vi "TypedescToEnum.vi"(1 "type desc":i16[](array[numeric])) -> (0 "DataType":u16)   [LabVIEW 2010]
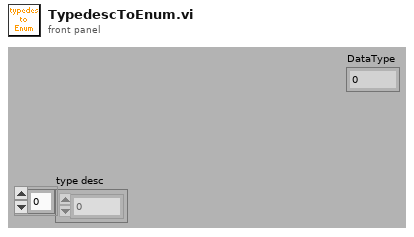
[diagram p1: front panel]
types:
  T1 = enum16{"I8", "I16", "I32", "U8", "U16", "U32", "SGL", "DBL", "Boolean", "String", "Array1D(I8)", "Array1D(I16)", "Array1D(I32)", "Array1D(U8)", "Array1D(U16)", "Array1D(U32)", "Array1D(SGL)", "Array1D(DBL)", "Array1D(Boolean)", "Array1D(String)", "Array2D(I8)", "Array2D(I16)", "Array2D(I32)", "Array2D(U8)", "Array2D(U16)", "Array2D(U32)", "Array2D(SGL)", "Array2D(DBL)", "Array2D(Boolean)", "Array2D(String)"}
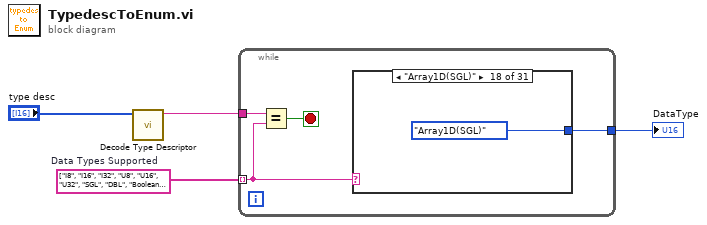
[diagram p0: block diagram]
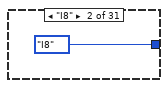
[diagram p3: hidden frame]
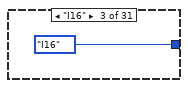
[diagram p4: hidden frame]
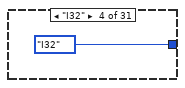
[diagram p5: hidden frame]
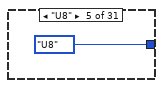
[diagram p6: hidden frame]
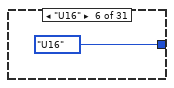
[diagram p7: hidden frame]
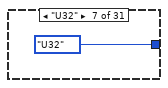
[diagram p8: hidden frame]
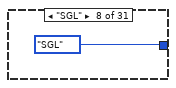
[diagram p9: hidden frame]
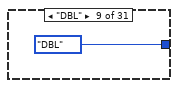
[diagram p10: hidden frame]
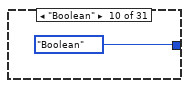
[diagram p11: hidden frame]
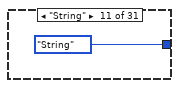
[diagram p12: hidden frame]
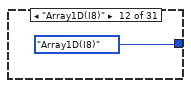
[diagram p13: hidden frame]
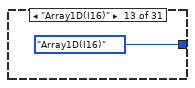
[diagram p14: hidden frame]
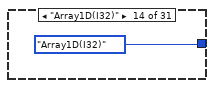
[diagram p15: hidden frame]
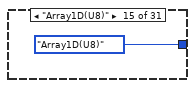
[diagram p16: hidden frame]
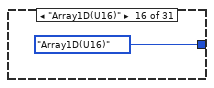
[diagram p17: hidden frame]
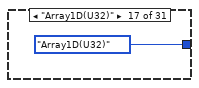
[diagram p18: hidden frame]
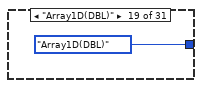
[diagram p19: hidden frame]
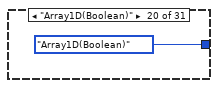
[diagram p20: hidden frame]
diagram:
  w3 = string[] ["I8", "I16", "I32", "U8", "U16", "U32", "SGL", "DBL", "Boolean", "String", "Array1D(I8)", "Array1D(I16)", "Array1D(I32)", "Array1D(U8)", "Array1D(U16)", "Array1D(U32)", "Array1D(SGL)", "Array1D(DBL)", "Array1D(Boolean)", "Array1D(String)", "Array2D(I8)", "Array2D(I16)", "Array2D(I32)", "Array2D(U8)", "Array2D(U16)", "Array2D(U32)", "Array2D(SGL)", "Array2D(DBL)", "Array2D(Boolean)", "Array2D(String)"]  # Data Types Supported
  n1 = call "Decode Type Descriptor.vi"("TypeDesc"="type desc") -> ("Type String"=w2:string)  [unwired: 1 in, 5 out]
  n2 = while {
    tunnel: w3 -> [w5] mode=indexing
    tunnel: w2 -> [w8]
    tunnel: [w6] -> w4
    stop <- w7 stop-if-true
    n3 = Equal?(x=w8, y=w5) -> (x = y?=w7:bool)
    n4 = case shown="\"Array1D(SGL)\"" w5 {
      tunnel: [_ T1."I8" ("DataType") T1."I16" ("DataType") T1."I32" ("DataType") T1."U8" ("DataType") T1."U16" ("DataType") T1."U32" ("DataType") T1."SGL" ("DataType") T1."DBL" ("DataType") T1."Boolean" ("DataType") T1."String" ("DataType") T1."Array1D(I8)" ("DataType") T1."Array1D(I16)" ("DataType") T1."Array1D(I32)" ("DataType") T1."Array1D(U8)" ("DataType") T1."Array1D(U16)" ("DataType") T1."Array1D(U32)" ("DataType") T1."Array1D(SGL)" ("DataType") T1."Array1D(DBL)" ("DataType") T1."Array1D(Boolean)" ("DataType") T1."Array1D(String)" ("DataType") T1."Array2D(I8)" ("DataType") T1."Array2D(I16)" ("DataType") T1."Array2D(I32)" ("DataType") T1."Array2D(U8)" ("DataType") T1."Array2D(U16)" ("DataType") T1."Array2D(U32)" ("DataType") T1."Array2D(SGL)" ("DataType") T1."Array2D(DBL)" ("DataType") T1."Array2D(Boolean)" ("DataType") T1."Array2D(String)" ("DataType")] -> w6
      frame Default {
      }
      frame "I8" {
      }
      frame "I16" {
      }
      frame "I32" {
      }
      frame "U8" {
      }
      frame "U16" {
      }
      frame "U32" {
      }
      frame "SGL" {
      }
      frame "DBL" {
      }
      frame "Boolean" {
      }
      frame "String" {
      }
      frame "Array1D(I8)" {
      }
      frame "Array1D(I16)" {
      }
      frame "Array1D(I32)" {
      }
      frame "Array1D(U8)" {
      }
      frame "Array1D(U16)" {
      }
      frame "Array1D(U32)" {
      }
      frame "Array1D(SGL)" {
      }
      frame "Array1D(DBL)" {
      }
      frame "Array1D(Boolean)" {
      }
      frame "Array1D(String)" {
      }
      frame "Array2D(I8)" {
      }
      frame "Array2D(I16)" {
      }
      frame "Array2D(I32)" {
      }
      frame "Array2D(U8)" {
      }
      frame "Array2D(U16)" {
      }
      frame "Array2D(U32)" {
      }
      frame "Array2D(SGL)" {
      }
      frame "Array2D(DBL)" {
      }
      frame "Array2D(Boolean)" {
      }
      frame "Array2D(String)" {
      }
    }
  }
  "DataType" <- w4
